vi "CleanUp.vi"(8 "ErrorIn":errorcluster caption="Error In", 11 "ObjectIn":refnum<class "ButtonCollection.lvclass"> caption="Object In") -> (0 "ErrorOut":errorcluster caption="Error Out", 3 "ObjectOut":refnum<class "ButtonCollection.lvclass"> caption="Object Out")   [LabVIEW 2021, in "ButtonCollection.lvclass"]
uses:
  ButtonCollection.lvclass
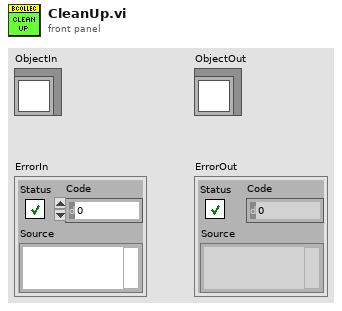
[diagram p1: front panel]
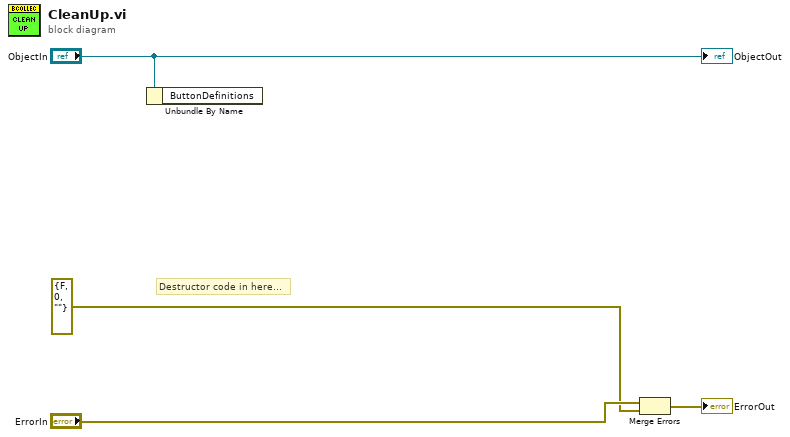
[diagram p0: block diagram]
diagram:
  # "Destructor code in here..."
  n1 = Unbundle By Name("ObjectIn") -> ()  [unwired: 1 out]
  n2 = Merge Errors("ErrorIn", errorcluster {"status"=FALSE, "code"=0, "source"=""} ("error in (no error)")) -> (→"ErrorOut":errorcluster)
  "ObjectOut" <- "ObjectIn"
